vi "Consulter_Bilan.vi"(0 "File Path 2":path) -> (1 "Date":string, 2 "Nombre de véhicules:":dbl, 3 "Nombre de \nvéhicules suspects:":dbl, 8 "Localisation":string, 10 "Image":T1(plugin-control))   [LabVIEW 2024]
uses:
  Assets/text_indicator.ctl
panel:
  in  "Consulter Bilan":bool
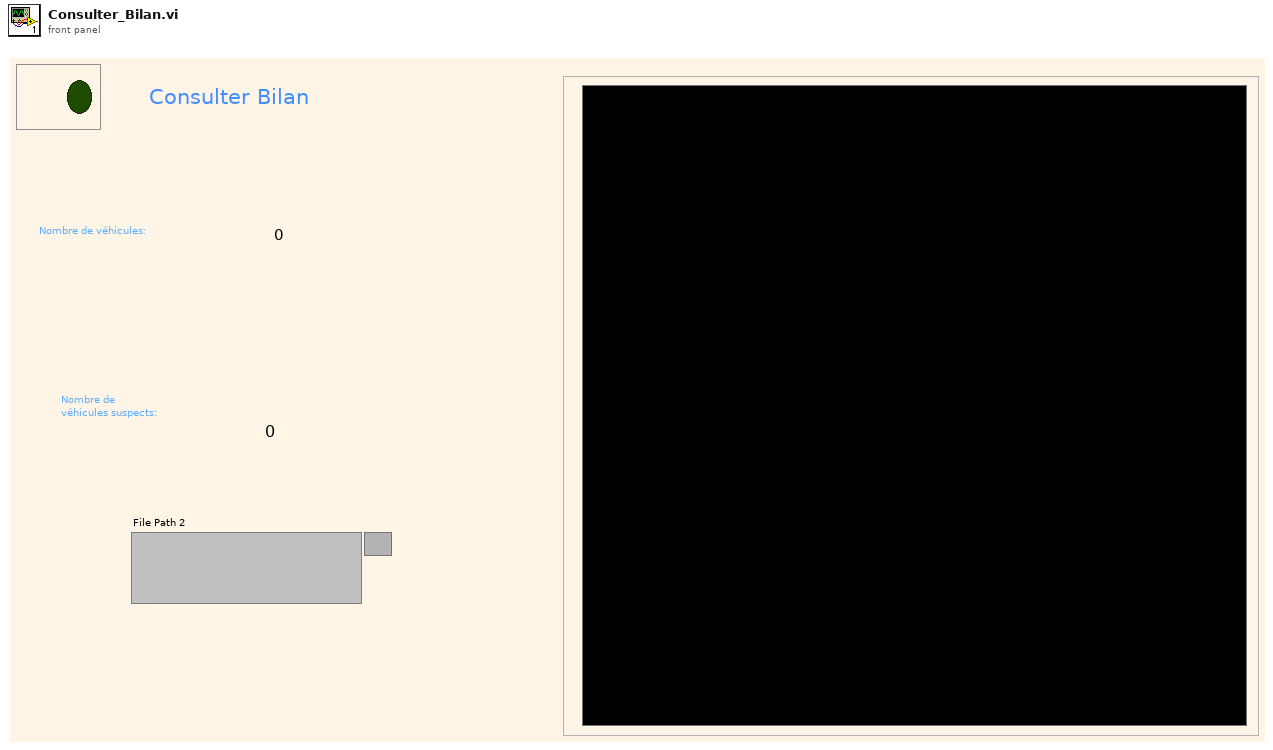
[diagram p1: front panel]
types:
  T1 = typedef "IMAQ Image.ctl" = refnum<image>
  T2 = typedef "Image Type" = u32
  T3 = typedef "text_indicator.ctl" = string
  T4 = cluster{"label":string, "confidence":i32, "detection_type":string, "bbox":dbl[], "crop_path":string, "vehicle_color":string}[]
  T5 = cluster{"Coordonnées\n Rectangles[0]":dbl, "Coordonnées\n Rectangles[1]":dbl, "Coordonnées\n Rectangles[2]":dbl, "Coordonnées\n Rectangles[3]":dbl}
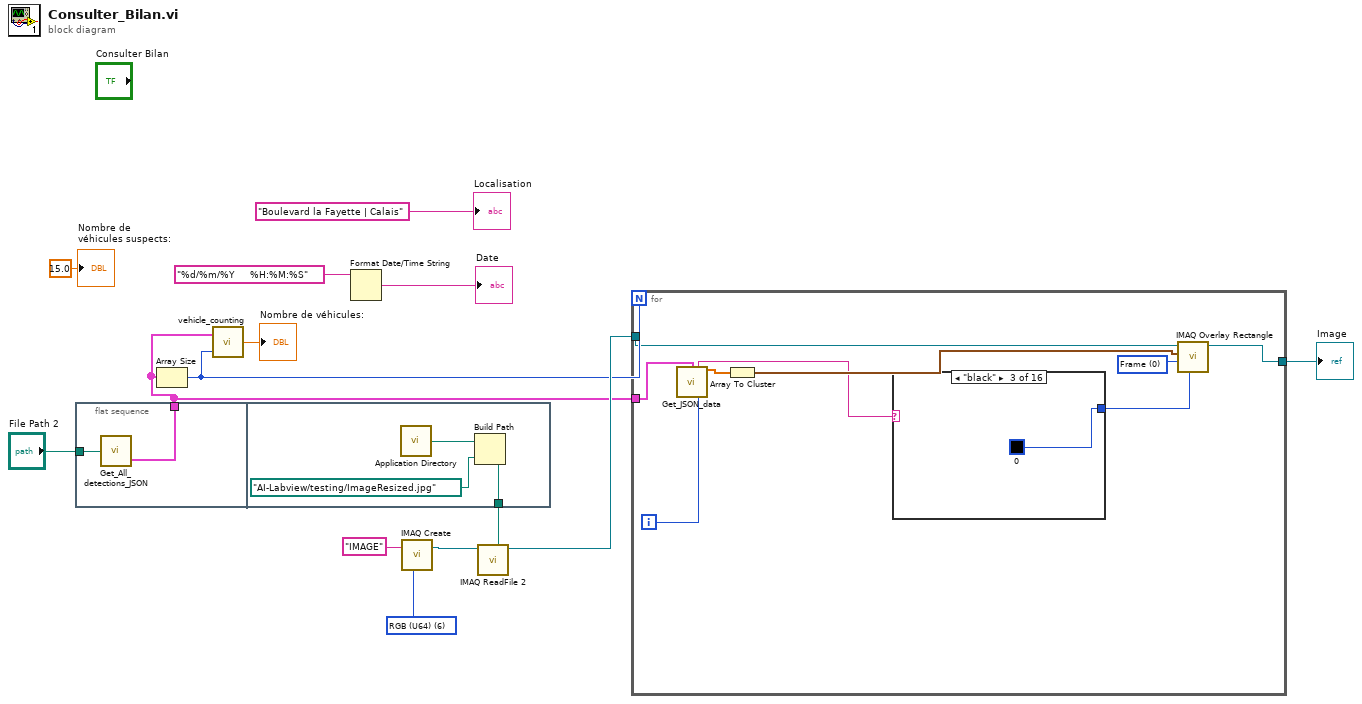
[diagram p0: block diagram]
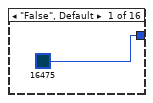
[diagram p2: hidden frame]
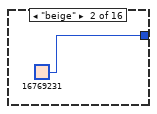
[diagram p3: hidden frame]
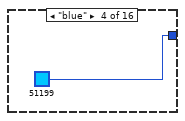
[diagram p4: hidden frame]
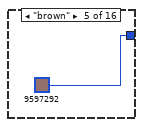
[diagram p5: hidden frame]
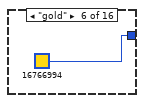
[diagram p6: hidden frame]
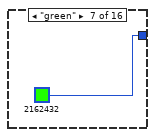
[diagram p7: hidden frame]
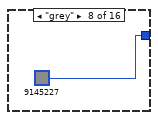
[diagram p8: hidden frame]
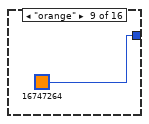
[diagram p9: hidden frame]
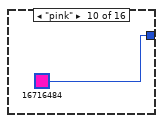
[diagram p10: hidden frame]
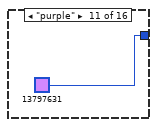
[diagram p11: hidden frame]
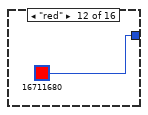
[diagram p12: hidden frame]
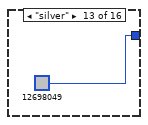
[diagram p13: hidden frame]
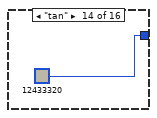
[diagram p14: hidden frame]
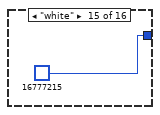
[diagram p15: hidden frame]
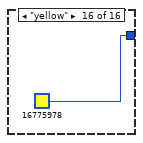
[diagram p16: hidden frame]
diagram:
  w12 = T2 6 items=["Grayscale (U8)", "Grayscale (I16)", "Grayscale (SGL)", "Complex (CSG)", "RGB (U32)", "HSL (U32)", "RGB (U64)", "Grayscale (U16)"] ("Image Type")
  n1 = flat-sequence {
    tunnel: [w16] -> w3
    tunnel: "File Path 2" -> [w15]
    tunnel: [w17] -> w7
    frame #0 {
      n2 = call "Get_All_detections_JSON.vi"("path"=w15) -> ("detections"=w16:T4)  [unwired: 4 in, 1 out]
    }
    frame #1 {
      n3 = call <vilib>:"Application Directory.vi"() -> ("Application Directory"=w19:path)
      n4 = Build Path(base path=w19, name or relative path=path "AI-Labview/testing/ImageResized.jpg") -> (appended path=w17:path)
    }
  }
  n5 = Array Size(array=w3) -> (size(s)=w2:i32)
  n6 = call "vehicle_counting.vi"("Size"=w2, "Array"=w3) -> ("Result"=→"Nombre de véhicules:":dbl)  [unwired: 1 in]
  n7 = Format Date/Time String(time format string (%c)="%d/%m/%Y     %H:%M:%S") -> (date/time string=→"Date":string)  [unwired: 2 in]
  n8 = call "IMAQ Create"("Image Name"="IMAGE", "Image Type"=w12) -> ("New Image"=w10:T1)  [unwired: 3 in, 1 out]
  n9 = call "IMAQ ReadFile 2"("File Path"=w7, "Image"=w10) -> ("Image Out"=w9:T1)  [unwired: 5 in, 4 out]
  n10 = for {
    N: w2 -> [_]
    tunnel: w9 -> [w27]
    tunnel: w3 -> [w23]
    tunnel: [w20] -> w4
    i -> [w25]
    w28 = u32 0 items=["Frame", "Fill", "Highlight"] ("Drawing Mode (Frame)")
    n11 = call "Get_JSON_data.vi"("array"=w23, "index\n detections"=w25) -> ("vehicle_color"=w22:string, "Coordonnées\n Rectangles"=w26:dbl[])  [unwired: 8 in, 4 out]
    n12 = Array To Cluster(array=w26) -> (cluster=w24:T5)
    n13 = case shown="\"black\"" w22 {
      tunnel: [u32 16475 ("Color") u32 16769231 ("Color") u32 0 ("Color") u32 51199 ("Color") u32 9597292 ("Color") u32 16766994 ("Color") u32 2162432 ("Color") u32 9145227 ("Color") u32 16747264 ("Color") u32 16716484 ("Color") u32 13797631 ("Color") u32 16711680 ("Color") u32 12698049 ("Color") u32 12433320 ("Color") u32 16777215 ("Color") u32 16775978 ("Color")] -> w21
      frame "False", Default {
      }
      frame "beige" {
      }
      frame "black" {
      }
      frame "blue" {
      }
      frame "brown" {
      }
      frame "gold" {
      }
      frame "green" {
      }
      frame "grey" {
      }
      frame "orange" {
      }
      frame "pink" {
      }
      frame "purple" {
      }
      frame "red" {
      }
      frame "silver" {
      }
      frame "tan" {
      }
      frame "white" {
      }
      frame "yellow" {
      }
    }
    n14 = call "IMAQ Overlay Rectangle"("Color"=w21, "Drawing Mode (Frame)"=w28, "Rectangle"=w24, "Image"=w27) -> ("Image Out"=w20:T1)  [unwired: 6 in, 1 out]
  }
  "Image" <- w4
  "Nombre de \nvéhicules suspects:" <- 15.0 ("Nombre de \nvéhicules suspects:")
  "Localisation" <- T3 "Boulevard la Fayette | Calais" ("Localisation")
